vi "GET_sensorID.vi"(8 "error in (no error)":errorcluster, 11 "Serial Number":string) -> (0 "error out":errorcluster, 3 "Sensor Data out":T1)   [LabVIEW 2018, in "MySQLTools.lvlib"]
uses:
  MySQLTools.lvlib
  TypeDefs/Sensor Data.ctl
  <vilib>/addons/database/Auxilliary.llb/DB Tools Cursor Type.ctl
  <vilib>/addons/database/Connection.llb/Conn Execute.vi
  <vilib>/addons/database/Recordset.llb/Rec Fetch Recordset Data (R).vi
  <vilib>/addons/database/_DB Variant To Data/Database Variant To Data.xnode
  <vilib>/addons/database/NI_Database_API.lvlib
panel:
  in  "Sensor Data":T1
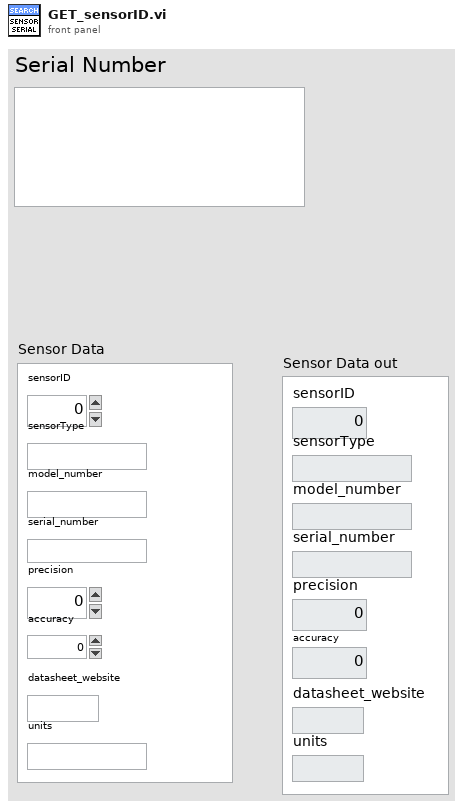
[diagram p1: front panel]
types:
  T1 = typedef "MySQLTools.lvlib/Sensor Data.ctl" = cluster{"sensorID":u16, "sensorType":string, "model_number":string, "serial_number":string, "precision":dbl, "accuracy":dbl, "datasheet_website":string, "units":string}
  T2 = typedef "NI_Database_API.lvlib/DB Tools Cursor Type.ctl" = enum16{"forward-only", "keyset", "dynamic", "static"}
  T3 = typedef "NI_Database_API.lvlib/Conn ObjectReference.ctl" = refnum<k1>
  T4 = typedef "NI_Database_API.lvlib/Rec ObjectReference.ctl" = refnum<k1>
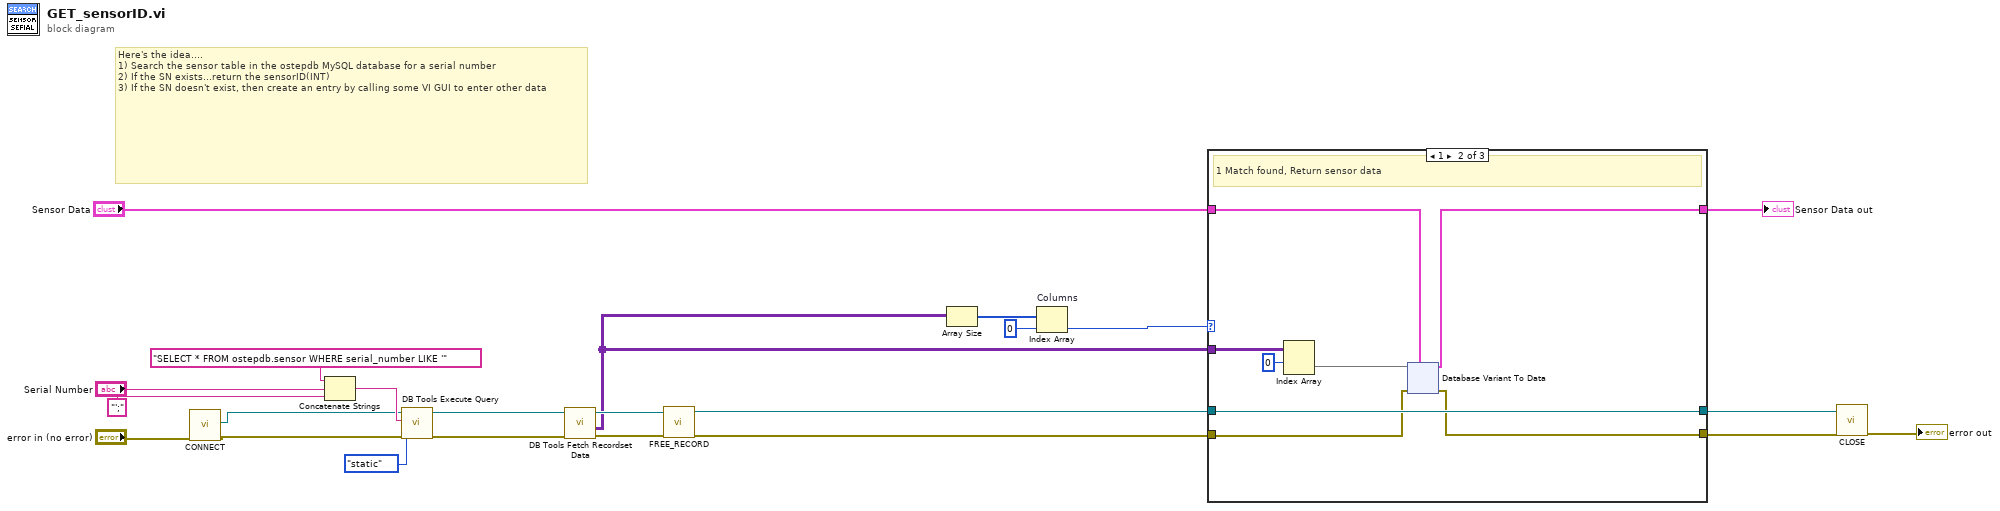
[diagram p0: block diagram]
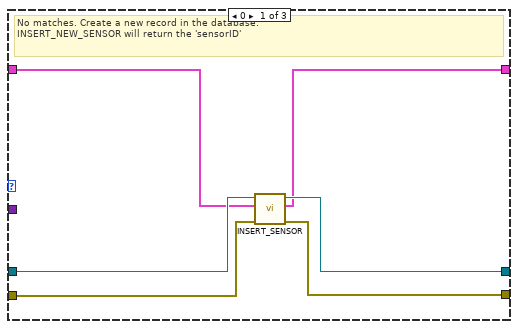
[diagram p2: hidden frame]
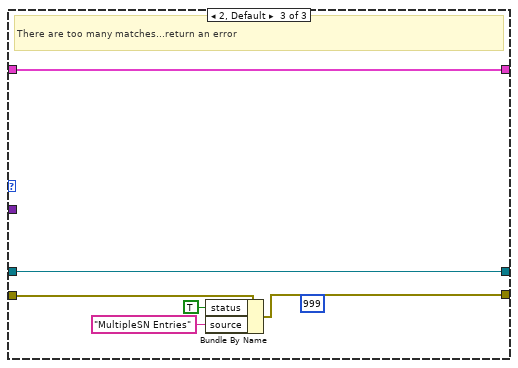
[diagram p3: hidden frame]
diagram:
  # "Here's the idea....\n1) Search the sensor table in the ostepdb MySQL database for a serial number\n2) If the SN exists...return the sensorID(INT)\n3) If the SN doesn't exist, then create an entry by calling some VI GUI to enter other data"
  n1 = call "CONNECT.vi"("error in (no error)"="error in (no error)") -> ("error out"=w22:errorcluster, "connection ref out"=w5:T3)  [unwired: 9 in]
  n2 = Concatenate Strings("SELECT * FROM ostepdb.sensor WHERE serial_number LIKE '" ("SQL query"), "Serial Number", "';" ("SQL query")) -> (w16:string)
  n3 = call-poly <vilib>:"DB Tools Execute Query.vi"("error in (no error)"=w22, "cursor type"=DB_Tools_Cursor_Type."static", "SQL query"=w16, "connection reference"=w5) -> ("error out"=w19:errorcluster, "recordset reference"=w20:T4)  [unwired: 4 in]
  n4 = call-poly <vilib>:"DB Tools Fetch Recordset Data.vi"("error in (no error)"=w19, "recordset reference"=w20) -> ("error out"=w14:errorcluster, "recordset data"=w13:variant[][], "recordset reference out"=w15:T4)  [unwired: 3 in]
  n5 = call "FREE_RECORD.vi"("error in (no error)"=w14, "Recordset Ref In"=w15) -> ("error out"=w9:errorcluster, "connection ref Out"=w4:T3)  [unwired: 8 in]
  n6 = Array Size(array=w13) -> (size(s)=w11:i32[])
  n7 = Index Array "Columns"(array=w11, index=0 ("disabled index (col)")) -> (element=w10:i32)
  n8 = case shown="1" w10 {
    tunnel: w9 -> [w29 w31 w295]
    tunnel: [w28 w30 w292] -> w8
    tunnel: w13 -> [_ w36 _]
    tunnel: w4 -> [w26 w37 w291]
    tunnel: [w27 w37 w291] -> w6
    tunnel: "Sensor Data" -> [w25 w33 w290]
    tunnel: [w24 w32 w290] -> w1
    frame 0 {
      # "No matches. Create a new record in the database.\nINSERT_NEW_SENSOR will return the 'sensorID'"
      n9 = call "INSERT_SENSOR.vi"("error in (no error)"=w29, "Sensor Data in"=w25, "Refnum in"=w26) -> ("error out"=w28:errorcluster, "Sensor Data out"=w24:T1, "Refnum out"=w27:T3)  [unwired: 6 in]
    }
    frame 1 {
      # "1 Match found, Return sensor data"
      n10 = Index Array(array=w36, index (row)=0) -> (element=w34:variant[])  [unwired: 1 in]
      n11 = xnode "Database Variant To Data"("database variant"=w34, "error in (no error)"=w31, "type"=w33) -> ("data"=w32:T1, "error out"=w30:errorcluster)
    }
    frame 2, Default {
      (unwired) u16 999
      # "There are too many matches...return an error"
      n12 = Bundle By Name(cluster=w295, "status"=TRUE, "source"="MultipleSN Entries") -> (w292:errorcluster)
    }
  }
  "Sensor Data out" <- w1
  n13 = call "CLOSE.vi"("error in (no error)"=w8, "Database Ref In"=w6) -> ("error out"=→"error out":errorcluster)  [unwired: 9 in]
